vi "1C.1 Camera Interpreter.vi"() -> (0 "error out":errorcluster, 1 "Overhead Image":T4(plugin-control), 2 "Heading":T1 format="%05.1f", 3 "Boat Location":T2, 4 "Time Elapsed (s)\nSince Last Image":dbl)   [LabVIEW 2011]
uses:
  <vilib>/userdefined/High Color/IMAQdx.ctl
  2-RIO/2 Typedefs/UTM Location.ctl
  2-RIO/2 Typedefs/heading.ctl
  2-RIO/2 Typedefs/indicator LED.ctl
  2-RIO/2 Globals/2 Global.vi
  <vilib>/vision/driver/NI_Vision_Acquisition_Software.lvlib
panel:
  in  "Reset Camera":bool
  in  "Camera Selector":T3="cam0"
  # "(ignore UTM Zone \nand Hemisphere for \nRC boat)"
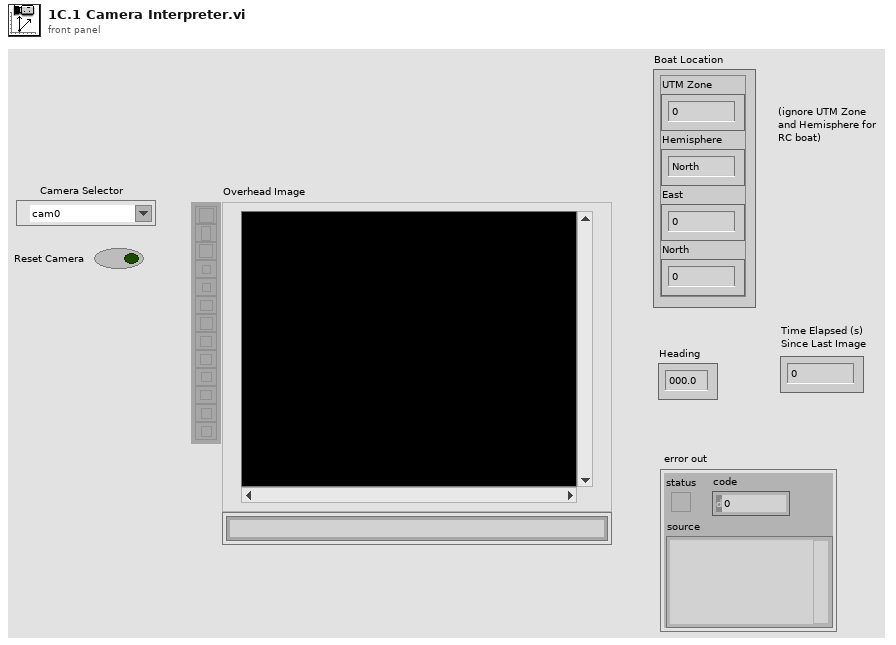
[diagram p1: front panel]
types:
  T1 = typedef "heading.ctl" = dbl
  T2 = typedef "UTM Location.ctl" = cluster{"UTM Zone":dbl, "Hemisphere":enum16{"North", "South"}, "East":dbl, "North":dbl}
  T3 = typedef "IMAQdx.ctl" = refnum<k21>
  T4 = typedef "IMAQ Image.ctl" = refnum<image>
  T5 = typedef "Image Type" = u32
  T6 = typedef "indicator LED.ctl" = bool
  T7 = typedef "generalized sensor status.ctl" = cluster{"Sensor Connected":T6, "Sensor Initialized":T6, "Sensor OK":T6, "Latest Error String":string}
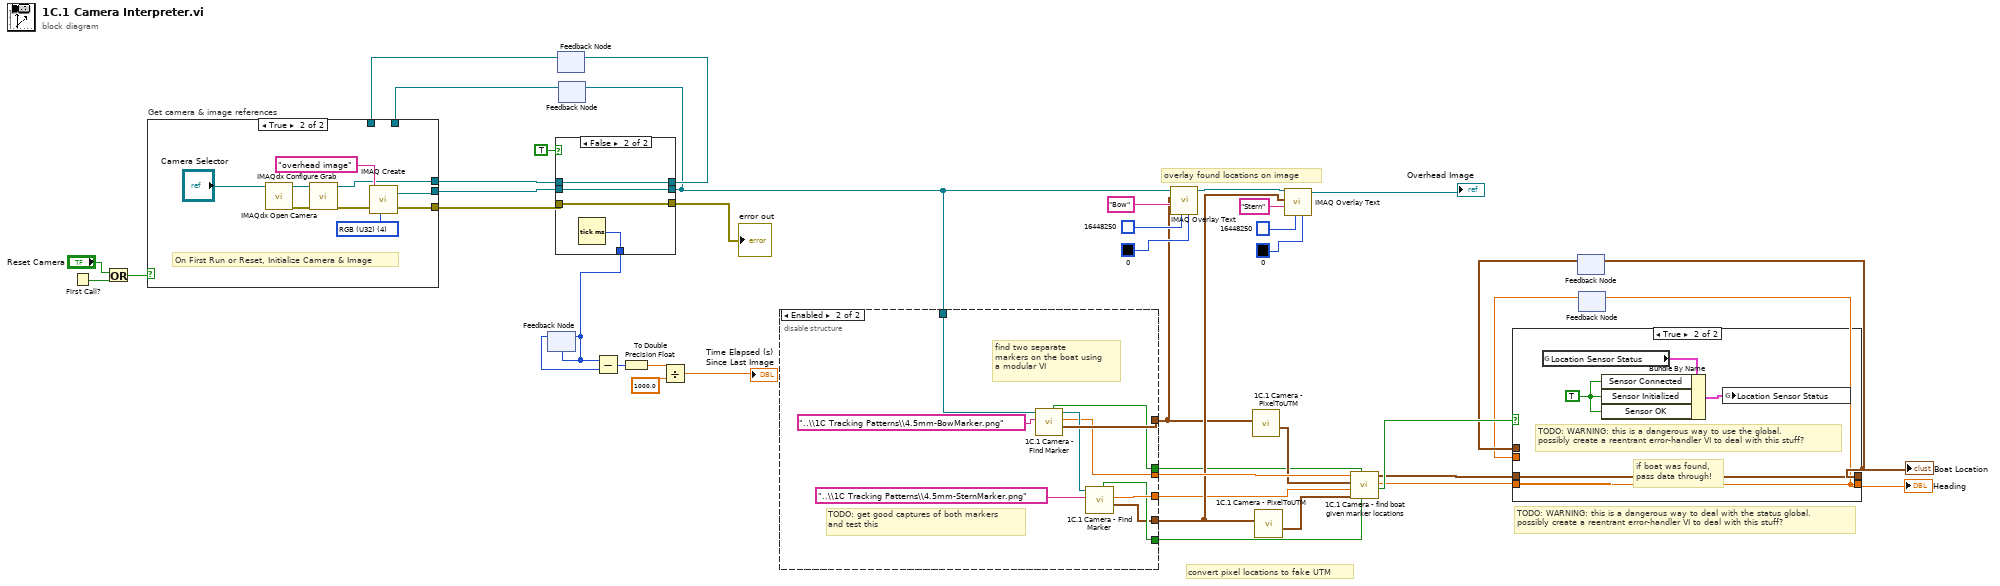
[diagram p0: block diagram]
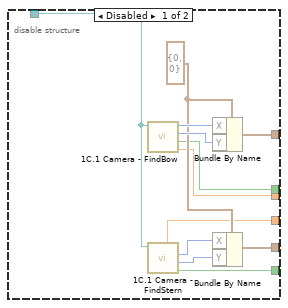
[diagram p2: hidden frame]
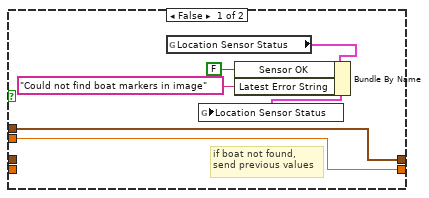
[diagram p3: hidden frame]
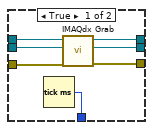
[diagram p4: hidden frame]
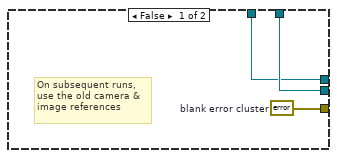
[diagram p5: hidden frame]
diagram:
  # "TODO: WARNING: this is a dangerous way to deal with the status global. \npossibly create a reentrant error-handler VI to deal with this stuff?"
  # "convert pixel locations to fake UTM"
  # "overlay found locations on image"
  n1 = First Call?() -> (First Call?: T/F=w40:bool)
  n2 = Or(x="Reset Camera", y=w40) -> (x .or. y?=w33:bool)
  n3 = feedback #1() -> (w34:T3)  [unwired: 1 in]
  n4 = feedback #2() -> (w35:T4)  [unwired: 1 in]
  n5 = case "Get camera & image references" shown="True" w33 {
    tunnel: [w43 w47] -> w39
    tunnel: [w42 w46] -> w38
    tunnel: [w44 w45] -> w37
    tunnel: w35 -> [w44 _]
    tunnel: w34 -> [w43 _]
    frame False {
      w42 = errorcluster {"status"=FALSE, "code"=0, "source"=""}  # blank error cluster
      # "On subsequent runs,\nuse the old camera &\nimage references"
    }
    frame True {
      w49 = T5 4 items=["Grayscale (U8)", "Grayscale (I16)", "Grayscale (SGL)", "Complex (CSG)", "RGB (U32)", "HSL (U32)", "RGB (U64)", "Grayscale (U16)"] ("Image Type")
      # "On First Run or Reset, Initialize Camera & Image"
      n6 = call <vilib>:"IMAQdx Open Camera.vi"("Session In"="Camera Selector") -> ("error out"=w50:errorcluster, "Session Out"=w53:T3)  [unwired: 9 in]
      n7 = call <vilib>:"IMAQdx Configure Grab.vi"("error in"=w50, "Session In"=w53) -> ("error out"=w51:errorcluster, "Session Out"=w47:T3)  [unwired: 8 in]
      n8 = call "IMAQ Create"("Image Name"="overhead image", "Image Type"=w49, "error in (no error)"=w51) -> ("New Image"=w45:T4, "error out"=w46:errorcluster)  [unwired: 2 in]
    }
  }
  n9 = case shown="False" TRUE {
    tunnel: [w60 w62] -> w41
    tunnel: w39 -> [w59 w64]
    tunnel: w38 -> [w58 w62]
    tunnel: w37 -> [w57 w63]
    tunnel: [w56 w63] -> w1
    tunnel: [w55 w64] -> w36
    tunnel: [w54 w61] -> w26
    frame True {
      n10 = Tick Count (ms)() -> (millisecond timer value=w54:u32)
      n11 = call <vilib>:"IMAQdx Grab.vi"("error in"=w58, "Image In"=w57, "Session In"=w59) -> ("error out"=w60:errorcluster, "Image Out"=w56:T4, "Session Out"=w55:T3)  [unwired: 5 in, 1 out]
    }
    frame False {
      n12 = Tick Count (ms)() -> (millisecond timer value=w61:u32)
    }
  }
  "error out" <- w41
  n13 = feedback-in #3(w26) -> ()
  n14 = feedback #3(w26) -> (w31:u32)
  n15 = feedback-in #1(w36) -> ()
  n16 = feedback-in #2(w1) -> ()
  n17 = Subtract(x=w26, y=w31) -> (x-y=w30:u32)
  n18 = To Double Precision Float(number=w30) -> (double precision float=w29:dbl)
  n19 = Divide(x=w29, y=1000.0) -> (x/y=→"Time Elapsed (s)\nSince Last Image":dbl)
  n20 = disable-structure shown="Enabled" {
    disable-tunnel: [w71 w83] -> w16
    disable-tunnel: [w70 w78] -> w15
    disable-tunnel: [w69 w85] -> w14
    disable-tunnel: [w68 w79] -> w12
    disable-tunnel: [w67 w77] -> w10
    disable-tunnel: [w66 w80] -> w9
    disable-tunnel: w1 -> [w65 w86]
    frame Disabled {
      w72 = cluster{"X":i32, "Y":i32} {"X"=0, "Y"=0} ("Origin")
      n21 = call "1C.1 Camera - FindBow.vi"("Refnum in"=w65) -> ("Bow Heading"=w71:T1, "Bow found?"=w67:T6, "bow pixel y"=w75:i32, "bow pixel x"=w76:i32)  [unwired: 7 in]
      n22 = call "1C.1 Camera - FindStern.vi"("Refnum in"=w65) -> ("Stern Found"=w68:T6, "y pixel"=w74:i32, "x pixel"=w73:i32, "Heading"=w66:T1)  [unwired: 6 in, 1 out]
      n23 = Bundle By Name(cluster=w72, "X"=w76, "Y"=w75) -> (w69:cluster{"X":i32, "Y":i32})
      n24 = Bundle By Name(cluster=w72, "X"=w73, "Y"=w74) -> (w70:cluster{"X":i32, "Y":i32})
    }
    frame Enabled {
      # "TODO: get good captures of both markers\nand test this"
      # "find two separate\nmarkers on the boat using \na modular VI"
      n25 = call "1C.1 Camera - Find Marker.vi"("marker template relative path"="..\\1C Tracking Patterns\\4.5mm-BowMarker.png", "Image In"=w86) -> ("Best Match Position"=w85:cluster{"x":sgl, "y":sgl}, "Best Match Heading"=w83:T1, "Image Out"=w84:T4, "Marker found?"=w77:T6)  [unwired: 5 in, 1 out]
      n26 = call "1C.1 Camera - Find Marker.vi"("marker template relative path"="..\\1C Tracking Patterns\\4.5mm-SternMarker.png", "Image In"=w84) -> ("Best Match Position"=w78:cluster{"x":sgl, "y":sgl}, "Best Match Heading"=w80:T1, "Marker found?"=w79:T6)  [unwired: 5 in, 2 out]
    }
  }
  n27 = call "IMAQ Overlay Text"("BG Color (Transparent)"=u32 0, "Text Color (black)"=u32 16448250, "String"="Bow", "Origin"=w14, "Image"=w1) -> ("Image Out"=w18:T4)  [unwired: 5 in, 1 out]
  n28 = call "1C.1 Camera - PixelToUTM.vi"("Found Marker Position in (pixels)"=w14) -> ("UTM Location Out"=w13:T2)  [unwired: 10 in]
  n29 = call "1C.1 Camera - PixelToUTM.vi"("Found Marker Position in (pixels)"=w15) -> ("UTM Location Out"=w11:T2)  [unwired: 10 in]
  n30 = call "IMAQ Overlay Text"("BG Color (Transparent)"=u32 0, "Text Color (black)"=u32 16448250, "String"="Stern", "Origin"=w15, "Image"=w18) -> ("Image Out"=→"Overhead Image":T4)  [unwired: 5 in, 1 out]
  n31 = call "1C.1 Camera - find boat given marker locations.vi"("Stern Marker Found"=w12, "Bow Marker Found"=w10, "Stern Marker Location"=w11, "Stern Marker Heading"=w9, "Bow Marker Location"=w13, "Bow Marker Heading"=w16) -> ("Boat Found"=w8:T6, "Heading"=w6:T1, "Boat Location"=w7:T2)  [unwired: 3 in]
  n32 = feedback #4() -> (w4:T2)  [unwired: 1 in]
  n33 = feedback #5() -> (w2:T1)  [unwired: 1 in]
  n34 = case shown="True" w8 {
    tunnel: [w92 w97] -> w5
    tunnel: w7 -> [_ w97]
    tunnel: [w91 w96] -> w3
    tunnel: w6 -> [_ w96]
    tunnel: w4 -> [w92 _]
    tunnel: w2 -> [w91 _]
    frame False {
      # "if boat not found,\nsend previous values"
      n35 = global read "2 Global.vi" "Location Sensor Status"() -> (w90:T7)
      n36 = Bundle By Name(cluster=w90, "Sensor OK"=T6 FALSE, "Latest Error String"="Could not find boat markers in image" ("Error String")) -> (w87:T7)
      n37 = global write "2 Global.vi" "Location Sensor Status"(w87) -> ()
    }
    frame True {
      w93 = T6 TRUE ("Sensor OK")
      # "TODO: WARNING: this is a dangerous way to use the global. \npossibly create a reentrant error-handler VI to deal with this stuff?"
      # "if boat was found, \npass data through!"
      n38 = global read "2 Global.vi" "Location Sensor Status"() -> (w95:T7)
      n39 = Bundle By Name(cluster=w95, "Sensor Connected"=w93, "Sensor Initialized"=w93, "Sensor OK"=w93) -> (w94:T7)
      n40 = global write "2 Global.vi" "Location Sensor Status"(w94) -> ()
    }
  }
  "Boat Location" <- w5
  "Heading" <- w3
  n41 = feedback-in #4(w5) -> ()
  n42 = feedback-in #5(w3) -> ()
